vi "HEWH Stable Test.vi"(1 "Equipment":T1={"COM Port"="COM1", "MW100"="MW100", "AG34970"="A-34972A", "WT500"="WT500"}) -> (6 "T button?":bool)   [LabVIEW 2009]
uses:
  EquipReferences.ctl
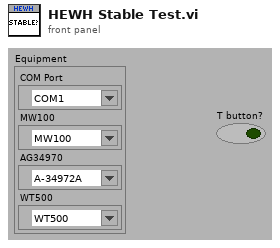
[diagram p1: front panel]
types:
  T1 = typedef "EquipReferences.ctl" = cluster{"COM Port":refnum<visa-resource-name>, "MW100":refnum<visa-resource-name>, "AG34970":refnum<visa-resource-name>, "WT500":refnum<visa-resource-name>}
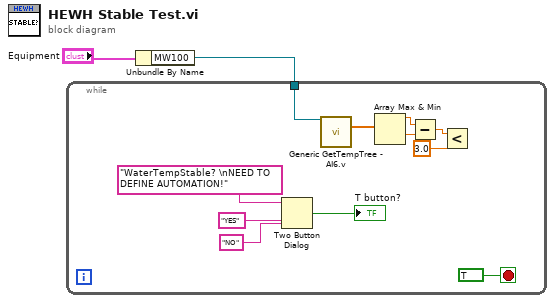
[diagram p0: block diagram]
diagram:
  n1 = Unbundle By Name("Equipment") -> ("MW100"=w1:refnum<visa-resource-name>)
  n2 = while {
    tunnel: w1 -> [w8]
    stop <- TRUE stop-if-true
    n3 = Two Button Dialog(message="WaterTempStable? \nNEED TO DEFINE AUTOMATION!", 1:"NO" ("F button name (\"Cancel\")"), 2:"YES" ("T button name (\"OK\")")) -> (T button?=→"T button?":bool)
    n4 = call "Generic GetTempTree - AI6.v.vi"("MW100"=w8) -> ("Tc Tree"=w7:dbl[])  [unwired: 12 in, 2 out]
    n5 = Array Max & Min(array=w7) -> (max value=w6:dbl, min value=w5:dbl)  [unwired: 2 out]
    n6 = Subtract(x=w6, y=w5) -> (x-y=w4:dbl)
    n7 = Less?(x=w4, y=3.0) -> ()  [unwired: 1 out]
  }
